vi "Init.vi"(0 "FrontPanelData in":refnum<class "EpiWrapper.lvclass">, 1 "MapPOS":refnum<vi>, 2 "Input":refnum<vi>, 3 "IntTime":i32=30000, 5 "MeasureControl":refnum<vi>, 9 "WaferTablle_Ref":refnum<vi>, 11 "error in (no error)":errorcluster, 12 "Wafer":refnum<vi>, 14 "INSTR_PARAM":refnum<vi>) -> (4 "FrontPanelData out":refnum<class "EpiWrapper.lvclass">, 15 "error out":errorcluster)   [LabVIEW 2012, in "EpiWrapper.lvclass"]
uses:
  EpiWrapper.lvclass
  Instruments.lvclass
  LotData.lvclass
  Controls/TestArea.ctl
  Controls/TestData.ctl
  Controls/MeasureControl.ctl
  Controls/USB4000_Data.ctl
  Controls/Instr_Param.ctl
  Controls/Config.ctl
panel:
  in  "ConfigRef":refnum<vi>
  # "Current Result"
  # "Measure Control"
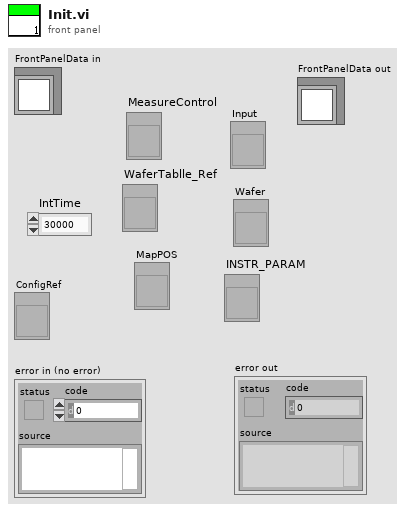
[diagram p1: front panel]
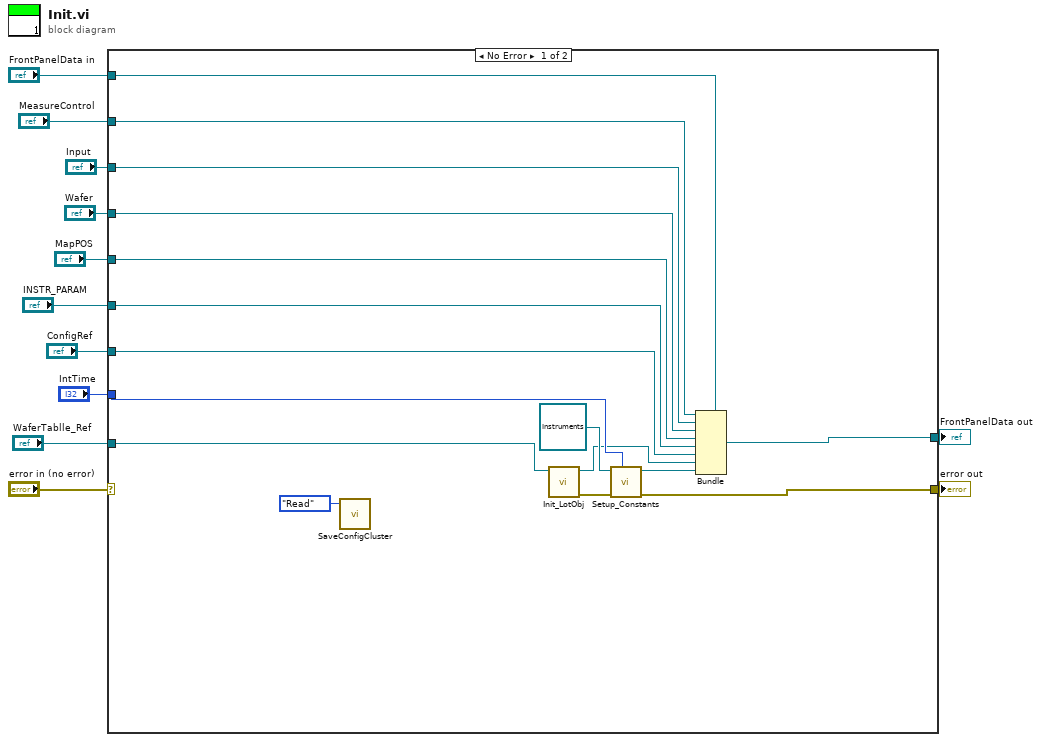
[diagram p0: block diagram]
diagram:
  n1 = case shown="No Error" "error in (no error)" {
    selector: "error in (no error)" -> [_ w30]
    tunnel: [w17 w30] -> w11
    tunnel: [w27 w29] -> w9
    tunnel: "FrontPanelData in" -> [w28 w29]
    tunnel: "WaferTablle_Ref" -> [w25 _]
    tunnel: "MeasureControl" -> [w22 _]
    tunnel: "Input" -> [w23 _]
    tunnel: "Wafer" -> [w21 _]
    tunnel: "MapPOS" -> [w20 _]
    tunnel: "INSTR_PARAM" -> [w19 _]
    tunnel: "IntTime" -> [w18 _]
    tunnel: "ConfigRef" -> [w16 _]
    frame No Error {
      n2 = call "SaveConfigCluster.vi"("Action"=enum16{"Read", "Write"}."Read") -> ()  [unwired: 2 in, 3 out]
      n3 = call "Init_LotObj.vi"("WaferTablle_Ref"=w25) -> ("error out"=w24:errorcluster, "LotData out"=w15:refnum<class "LotData.lvclass">)  [unwired: 9 in]
      n4 = call-dynamic "Setup_Constants.vi"("IntTime"=w18, "error in (no error)"=w24, "Instruments in"=refnum<class "Instruments.lvclass"> refnum ("Instruments.lvclass")) -> ("error out"=w17:errorcluster, "Instruments out"=w14:refnum<class "Instruments.lvclass">)  [unwired: 7 in]
      n5 = Bundle(cluster=w28, w22, w23, w21, w20, w19, w16, w15, w14) -> (w27:refnum<class "EpiWrapper.lvclass">)
    }
    frame Error {
    }
  }
  "error out" <- w11
  "FrontPanelData out" <- w9
